vi "from string.vi"(8 "error in":errorcluster, 9 "data":string, 10 "version":string, 11 "Standard Engine Repo Data in":refnum<class "synchronous engine configuration.lvclass">) -> (0 "error out":errorcluster, 3 "Standard Engine Repo Data out":refnum<class "synchronous engine configuration.lvclass">)   [LabVIEW 2013, in "synchronous engine configuration.lvclass"]
uses:
  synchronous engine configuration.lvclass
  Engine Configuration/engine configuration.lvclass
  synchronous engine configuration.lvclass/synchronous engine configuration.ctl
  <vilib>/NI/Tag Bus Module Framework/root configuration/TBM configuration.lvclass
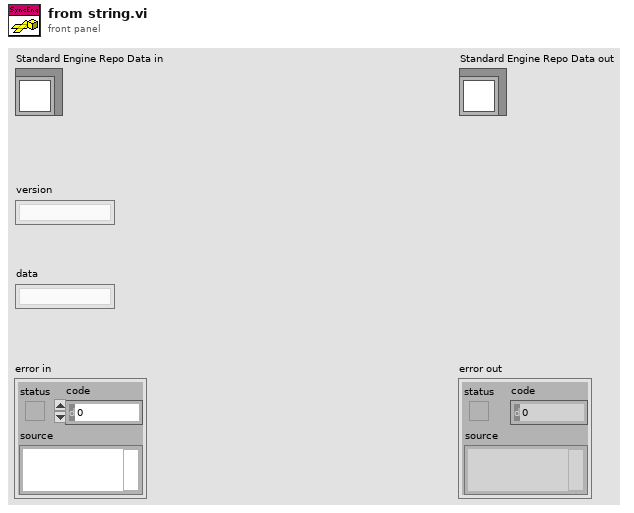
[diagram p1: front panel]
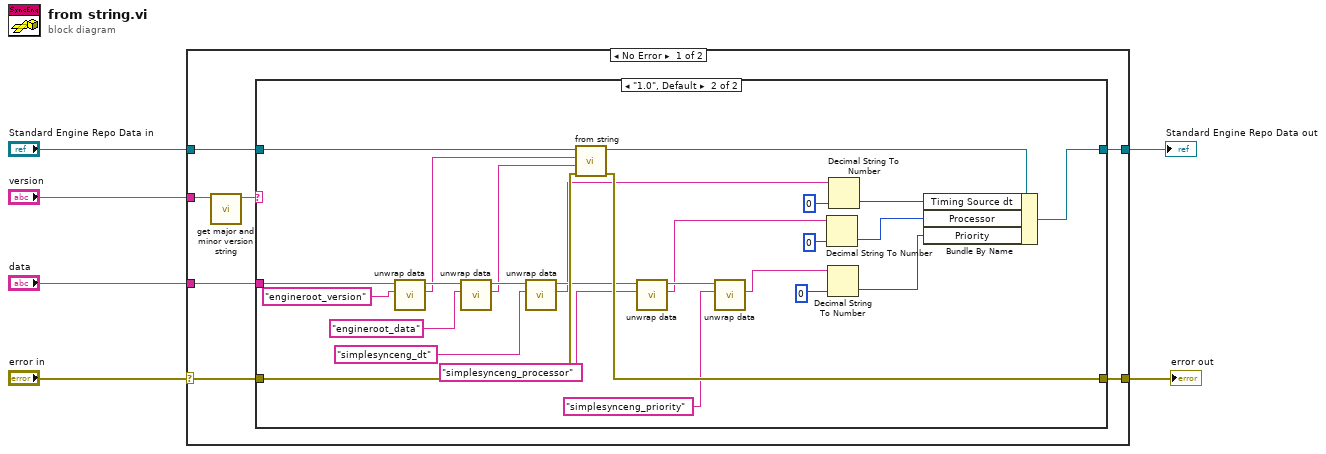
[diagram p0: block diagram]
diagram:
  n1 = case shown="No Error" "error in" {
    selector: "error in" -> [w7 w42]
    tunnel: [w13 w42] -> w6
    tunnel: [w12 w43] -> w5
    tunnel: "data" -> [w11 _]
    tunnel: "Standard Engine Repo Data in" -> [w10 w43]
    tunnel: "version" -> [w9 _]
    frame No Error {
      n2 = call <vilib>:"get major and minor version string.vi"("full version"=w9) -> ("major.minor version"=w8:string)  [unwired: 10 in]
      n3 = case shown="\"1.0\", Default" w8 {
        tunnel: w7 -> [w14 w41]
        tunnel: [w14 w40] -> w13
        tunnel: [w15 w39] -> w12
        tunnel: w11 -> [_ w31]
        tunnel: w10 -> [w15 w38]
        frame "False" {
        }
        frame "1.0", Default {
          n4 = call <vilib>:"unwrap data.vi"("identifier"="engineroot_version" ("additional identifier"), "data to unwrap"=w31) -> ("unwrapped data"=w30:string, "remaining string"=w32:string)  [unwired: 8 in]
          n5 = call <vilib>:"unwrap data.vi"("identifier"="engineroot_data" ("additional identifier"), "data to unwrap"=w32) -> ("unwrapped data"=w29:string, "remaining string"=w35:string)  [unwired: 8 in]
          n6 = call <vilib>:"unwrap data.vi"("identifier"="simplesynceng_dt" ("additional identifier"), "data to unwrap"=w35) -> ("unwrapped data"=w22:string, "remaining string"=w27:string)  [unwired: 8 in]
          n7 = call-parent "from string.vi"("error in"=w41, "data"=w29, "version"=w30, "engine configuration in"=w38) -> ("error out"=w40:errorcluster, "engine configuration out"=w37:refnum<class "synchronous engine configuration.lvclass">)  [unwired: 6 in]
          n8 = call <vilib>:"unwrap data.vi"("identifier"="simplesynceng_processor" ("additional identifier"), "data to unwrap"=w27) -> ("unwrapped data"=w23:string, "remaining string"=w28:string)  [unwired: 8 in]
          n9 = call <vilib>:"unwrap data.vi"("identifier"="simplesynceng_priority" ("additional identifier"), "data to unwrap"=w28) -> ("unwrapped data"=w24:string)  [unwired: 8 in, 1 out]
          n10 = Decimal String To Number(string=w23, default (0L)=0 ("Priority")) -> (number=w20:i32)  [unwired: 1 in, 1 out]
          n11 = Decimal String To Number(string=w24, default (0L)=0 ("Processor")) -> (number=w19:i32)  [unwired: 1 in, 1 out]
          n12 = Decimal String To Number(string=w22, default (0L)=u32 0 ("Timing Source dt")) -> (number=w21:u32)  [unwired: 1 in, 1 out]
          n13 = Bundle By Name(cluster=w37, "Timing Source dt"=w21, "Processor"=w20, "Priority"=w19) -> (w39:refnum<class "synchronous engine configuration.lvclass">)
        }
      }
    }
    frame Error {
    }
  }
  "error out" <- w6
  "Standard Engine Repo Data out" <- w5
